vi "Get Listbox Item.vi"(8 "error in (no error)":errorcluster) -> (0 "error out":errorcluster, 2 "OK?":bool, 3 "Item out":string)   [LabVIEW 2018, in "Instrument Addon System Explorer.lvlib"]
uses:
  Instrument Addon System Explorer.lvlib
panel:
  in  "Cancel":bool
  in  "OK":bool
  in  "New Item":string
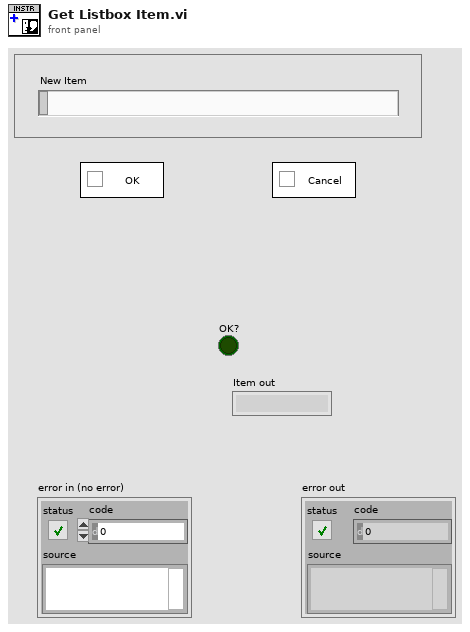
[diagram p1: front panel]
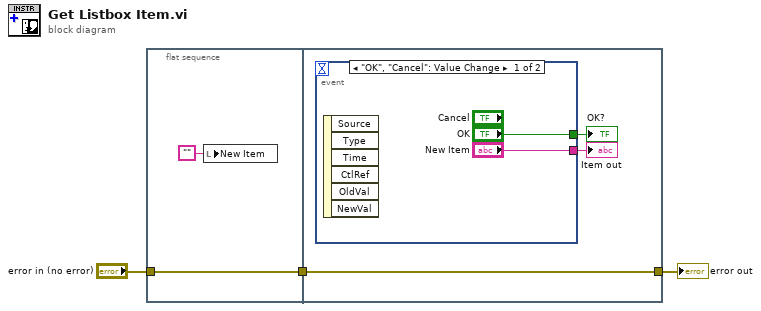
[diagram p0: block diagram]
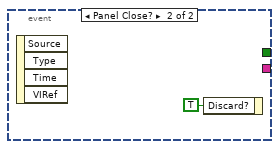
[diagram p2: hidden frame]
diagram:
  n1 = flat-sequence {
    tunnel: [w4] -> w2
    tunnel: "error in (no error)" -> [w4]
    tunnel: [w6] -> w3
    tunnel: w2 -> [w6]
    frame #0 {
      n2 = local write "New Item"("") -> ()
    }
    frame #1 {
      n3 = event shown="[0] \"OK\", \"Cancel\": Value Change" {
        selector: _ -> [_ _]
        dyn-events: _ -> [_ _]
        timeout: _ -> [_ _]
        tunnel: ["OK" _] -> w8
        tunnel: ["New Item" _] -> w7
        event "OK", "Cancel": Value Change {
          n4 = event-data() -> ()  [unwired: 1 in, 6 out]
        }
        event Panel Close? {
          n5 = event-data() -> ()  [unwired: 1 in, 4 out]
          n6 = event-data("Discard?"=TRUE) -> ()  [unwired: 1 in, 1 out]
        }
      }
      "OK?" <- w8
      "Item out" <- w7
    }
  }
  "error out" <- w3
